vi "Camera_ColorSegmentation.vi"(8 "error in (no error)":errorcluster, 10 "Bins":enum16{"Zero all", "1", "2", "3", "4"}(ring), 11 "SRV In":refnum<k5>) -> (0 "error out":errorcluster, 3 "SRV Out":refnum<k5>)   [LabVIEW 2014]
doc: "Set up the camera segmentation.\n\n\nModified for Benilde St. Margaret's School - Tim Jump\nBy Doug Schmertman - Logic PD\nCopyright 2012"
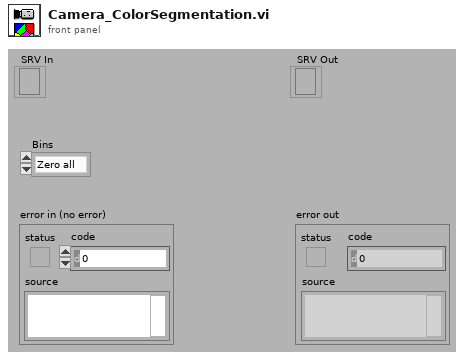
[diagram p1: front panel]
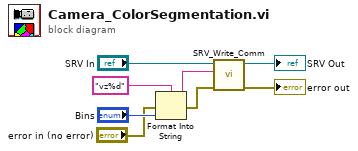
[diagram p0: block diagram]
diagram:
  n1 = Format Into String(format string="vz%d" ("Command Sent"), error in="error in (no error)", "Bins") -> (resulting string=w7:string, error out=w2:errorcluster)  [unwired: 1 in]
  n2 = call "SRV_Write_Comm.vi"("error in (no error)"=w2, "Command Sent"=w7, "SRV In"="SRV In") -> ("error out"=→"error out":errorcluster, "SRV Out"=→"SRV Out":refnum<k5>)  [unwired: 6 in, 1 out]
